vi "MICSD Reset Serial Port.vi"(8 "error in (no error)":errorcluster, 11 "VISA Resource Name":refnum<visa-resource-name>) -> (0 "error out":errorcluster, 3 "dup VISA Resource Name":refnum<visa-resource-name>)   [LabVIEW 2020]
uses:
  <vilib>/Instr/_visa.llb/VISA Configure Serial Port (Instr).vi
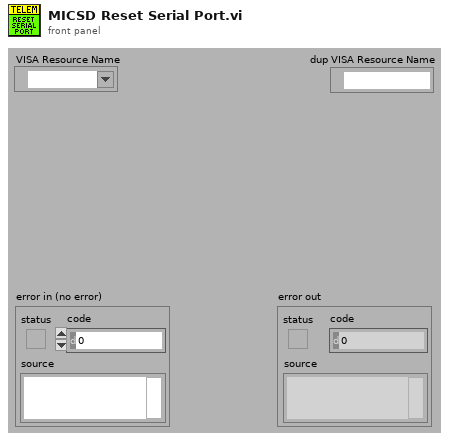
[diagram p1: front panel]
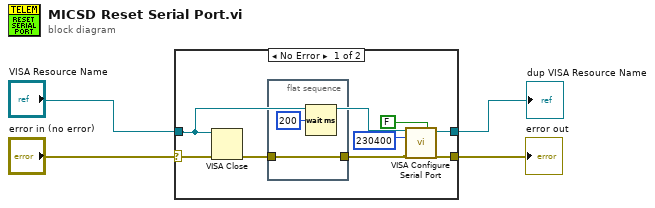
[diagram p0: block diagram]
diagram:
  n1 = case shown="No Error" "error in (no error)" {
    selector: "error in (no error)" -> [w8 w16]
    tunnel: [w10 w16] -> w3
    tunnel: "VISA Resource Name" -> [w7 w15]
    tunnel: [w9 w15] -> w4
    frame No Error {
      n2 = VISA Close(VISA resource name=w7, error in (no error)=w8) -> (error out=w6:errorcluster)
      n3 = flat-sequence {
        tunnel: w6 -> [w14]
        tunnel: [w14] -> w5
        frame #0 {
          n4 = Wait (ms)(milliseconds to wait=u32 200) -> ()  [unwired: 1 out]
        }
      }
      n5 = call-poly "VISA Configure Serial Port"("VISA resource name"=w7, "Enable Termination\nChar (T)"=FALSE ("Enable Termination\nChar (T)"), "baud rate (9600)"=u32 230400, "error in (no error)"=w5) -> ("VISA resource name out"=w9:refnum<visa-resource-name>, "error out"=w10:errorcluster)  [unwired: 10 in]
    }
    frame Error {
    }
  }
  "dup VISA Resource Name" <- w4
  "error out" <- w3
